vi "Pack PII Error_v00.vi"(8 "PII+Error Doubler":T4, 9 "PII+Error MCC":T4, 10 "PII+Error B":T4, 11 "PII+Error A":T4) -> (0 "Thresholds":T1, 3 "Error packed":T3={"Pre-Offset"={"Pre-Offset 1"=2, "Pre-Offset 2"=0, "Pre-Offset 3"=0, "Pre-Offset 4"=0, "Pre-Offset 5"=2, "Pre-Offset 6"=0, "Pre-Offset 7"=0, "Pre-Offset 8"=0}, "Post-Offset "={"Offset 1"=0, "Offset 2"=0, "Offset 3"=0, "Offset 4"=0, "Offset 5"=0, "Offset 6"=0, "Offset 7"=0, "Offset 8"=0}, "Gains"={"Gain 1"=0, "Gain 2"=0, "Gain 3"=0, "Gain 4"=0, "Gain 5"=0, "Gain 6"=0, "Gain 7"=0, "Gain 8"=0}, "Polarity DC"={"False 1"=FALSE, "False 2"=FALSE, "False 3"=FALSE, "False 4"=FALSE, "DC x -1"=FALSE, "DC x -1 2"=FALSE, "DC x -1 3"=FALSE, "DC x -1 4"=FALSE}})   [LabVIEW 2010]
doc: "Packages individual values related to error signal scaling from the user interface into data structures compatible with FPGA_Cavities.VI\n(very messy, could use a tidy)."
uses:
  Strict Type Defs/Error Scale.ctl
  Strict Type Defs/Controls Converted.ctl
  Strict Type Defs/Errors Converted.ctl
  Strict Type Defs/PII individual.ctl
panel:
  in  "Thresholds type def":T1
  in  "Re-Scan Thresh":T2
  in  "Lock Thresh":T2
  in  "Error scale FPGA type def":T3={"Pre-Offset"={"Pre-Offset 1"=0, "Pre-Offset 2"=300, "Pre-Offset 3"=0, "Pre-Offset 4"=0, "Pre-Offset 5"=0, "Pre-Offset 6"=0, "Pre-Offset 7"=0, "Pre-Offset 8"=0}, "Post-Offset "={"Offset 1"=0, "Offset 2"=300, "Offset 3"=0, "Offset 4"=0, "Offset 5"=0, "Offset 6"=0, "Offset 7"=0, "Offset 8"=0}, "Gains"={"Gain 1"=1, "Gain 2"=1, "Gain 3"=1, "Gain 4"=1, "Gain 5"=1, "Gain 6"=1, "Gain 7"=1, "Gain 8"=1}, "Polarity DC"={"False 1"=FALSE, "False 2"=FALSE, "False 3"=FALSE, "False 4"=FALSE, "DC x -1"=FALSE, "DC x -1 2"=FALSE, "DC x -1 3"=FALSE, "DC x -1 4"=FALSE}}
  in  "Polarity DC":T7
  in  "Pre Offset":T8
  in  "Offset":T9
  in  "Gains":T10
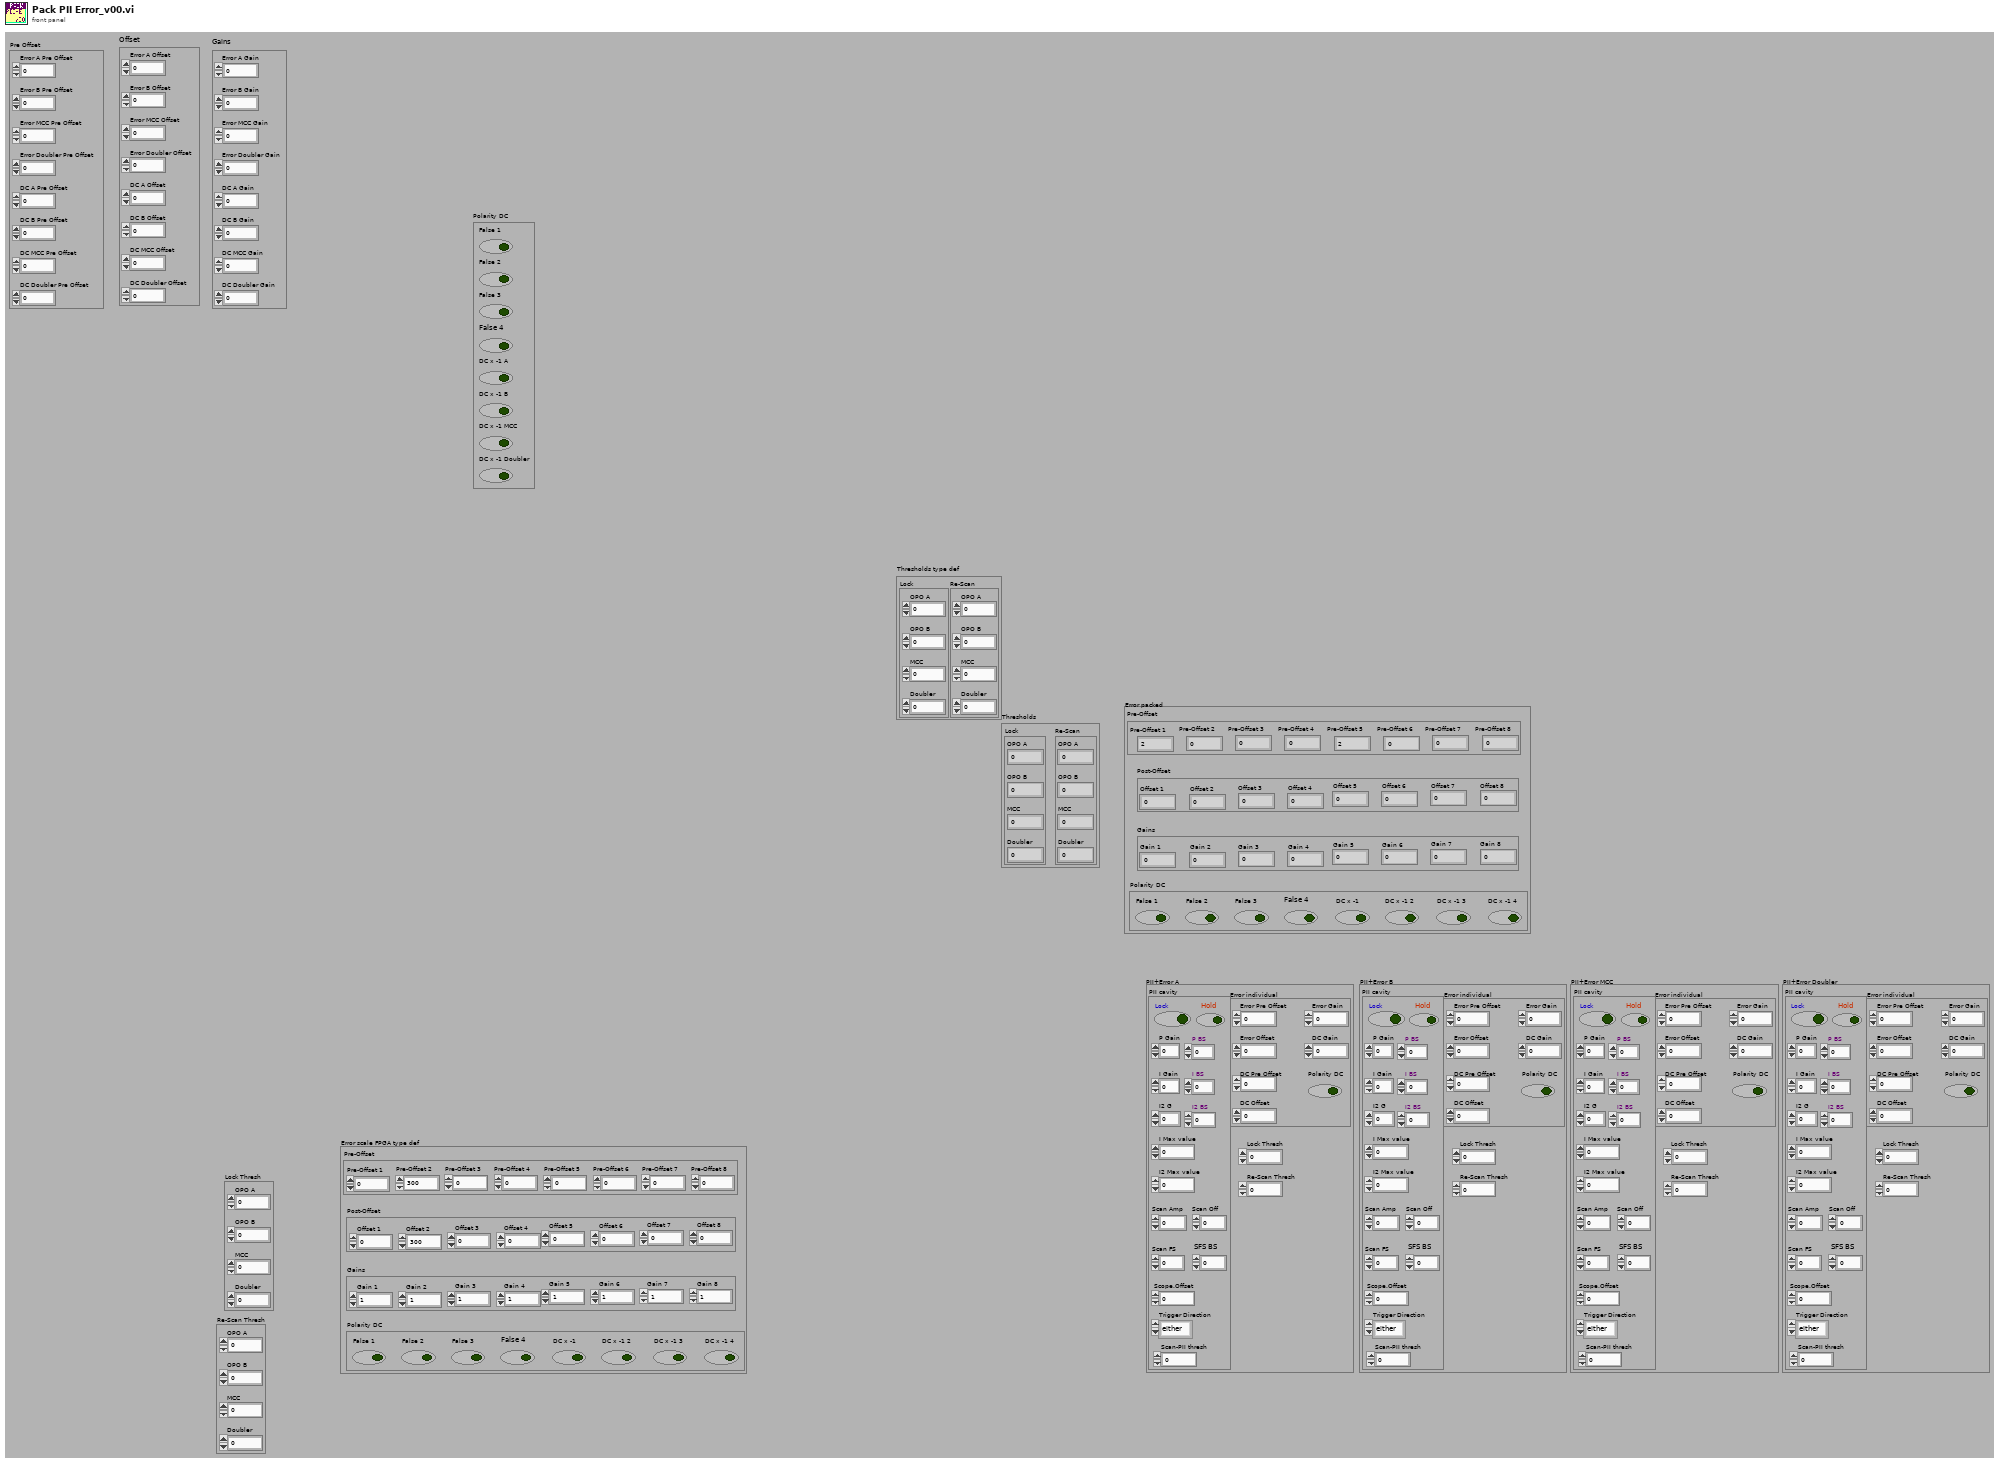
[diagram p1: front panel]
types:
  T1 = cluster{"Lock":cluster{"OPO A":i16, "OPO B":i16, "MCC":i16, "Doubler":i16}, "Re-Scan":cluster{"OPO A":i16, "OPO B":i16, "MCC":i16, "Doubler":i16}}
  T2 = cluster{"OPO A":i16, "OPO B":i16, "MCC":i16, "Doubler":i16}
  T3 = typedef "Error Scale.ctl" = cluster{"Pre-Offset":cluster{"Pre-Offset 1":i16, "Pre-Offset 2":i16, "Pre-Offset 3":i16, "Pre-Offset 4":i16, "Pre-Offset 5":i16, "Pre-Offset 6":i16, "Pre-Offset 7":i16, "Pre-Offset 8":i16}, "Post-Offset ":cluster{"Offset 1":i16, "Offset 2":i16, "Offset 3":i16, "Offset 4":i16, "Offset 5":i16, "Offset 6":i16, "Offset 7":i16, "Offset 8":i16}, "Gains":cluster{"Gain 1":i16, "Gain 2":i16, "Gain 3":i16, "Gain 4":i16, "Gain 5":i16, "Gain 6":i16, "Gain 7":i16, "Gain 8":i16}, "Polarity DC":cluster{"False 1":bool, "False 2":bool, "False 3":bool, "False 4":bool, "DC x -1":bool, "DC x -1 2":bool, "DC x -1 3":bool, "DC x -1 4":bool}}
  T4 = typedef "Controls Converted.ctl" = cluster{"Error individual":T5, "PII cavity":T6, "Lock Thresh":i16, "Re-Scan Thresh":i16}
  T5 = typedef "Errors Converted.ctl" = cluster{"Error Pre Offset":i16, "Error Offset":i16, "DC Pre Offset":i16, "DC Offset":i16, "Polarity DC":bool, "Error Gain":i16, "DC Gain":i16}
  T6 = typedef "PII individual.ctl" = cluster{"Lock":bool, "Hold":bool, "P Gain":i32, "P BS":i16, "I Gain":i32, "I BS":i16, "I2 G":i32, "I2 BS":i16, "Scan Amp":i16, "Scan Off":i16, "Scan FS":u16, "SFS BS":i16, "I Max value":i32, "I2 Max value":i32, "Scope.Offset":i16, "Trigger Direction":enum8{"either", "minus-plus", "plus-minus"}, "Scan-PII thresh":i16}
  T7 = cluster{"False 1":bool, "False 2":bool, "False 3":bool, "False 4":bool, "DC x -1 A":bool, "DC x -1 B":bool, "DC x -1 MCC":bool, "DC x -1 Doubler":bool}
  T8 = cluster{"Error A Pre Offset":i16, "Error B Pre Offset":i16, "Error MCC Pre Offset":i16, "Error Doubler Pre Offset":i16, "DC A Pre Offset":i16, "DC B Pre Offset":i16, "DC MCC Pre Offset":i16, "DC Doubler Pre Offset":i16}
  T9 = cluster{"Error A Offset":i16, "Error B Offset":i16, "Error MCC Offset":i16, "Error Doubler Offset":i16, "DC A Offset":i16, "DC B Offset":i16, "DC MCC Offset":i16, "DC Doubler Offset":i16}
  T10 = cluster{"Error A Gain":i16, "Error B Gain":i16, "Error MCC Gain":i16, "Error Doubler Gain":i16, "DC A Gain":i16, "DC B Gain":i16, "DC MCC Gain":i16, "DC Doubler Gain":i16}
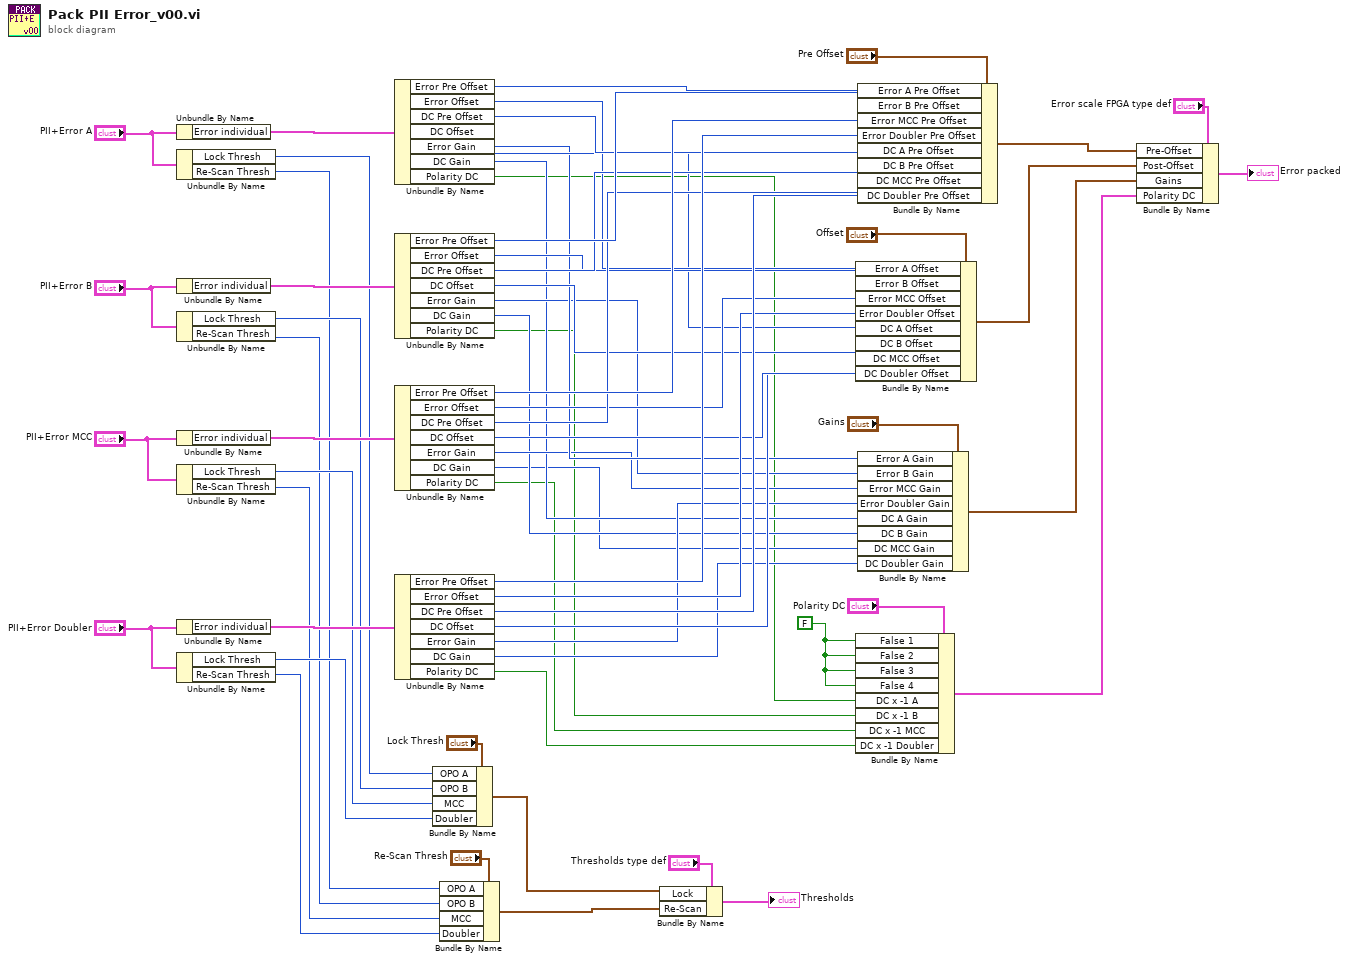
[diagram p0: block diagram]
diagram:
  w27 = FALSE ("False 1")
  n1 = Unbundle By Name("PII+Error A") -> ("Error individual"=w60:T5)
  n2 = Unbundle By Name("PII+Error A") -> ("Lock Thresh"=w13:i16, "Re-Scan Thresh"=w8:i16)
  n3 = Unbundle By Name("PII+Error B") -> ("Error individual"=w59:T5)
  n4 = Unbundle By Name("PII+Error B") -> ("Lock Thresh"=w12:i16, "Re-Scan Thresh"=w7:i16)
  n5 = Unbundle By Name("PII+Error MCC") -> ("Error individual"=w57:T5)
  n6 = Unbundle By Name("PII+Error MCC") -> ("Lock Thresh"=w11:i16, "Re-Scan Thresh"=w6:i16)
  n7 = Unbundle By Name("PII+Error Doubler") -> ("Error individual"=w58:T5)
  n8 = Unbundle By Name("PII+Error Doubler") -> ("Lock Thresh"=w10:i16, "Re-Scan Thresh"=w5:i16)
  n9 = Unbundle By Name(w60) -> ("Error Pre Offset"=w55:i16, "Error Offset"=w47:i16, "DC Pre Offset"=w51:i16, "DC Offset"=w43:i16, "Error Gain"=w39:i16, "DC Gain"=w35:i16, "Polarity DC"=w31:bool)
  n10 = Unbundle By Name(w59) -> ("Error Pre Offset"=w54:i16, "Error Offset"=w46:i16, "DC Pre Offset"=w50:i16, "DC Offset"=w42:i16, "Error Gain"=w38:i16, "DC Gain"=w34:i16, "Polarity DC"=w30:bool)
  n11 = Unbundle By Name(w57) -> ("Error Pre Offset"=w53:i16, "Error Offset"=w45:i16, "DC Pre Offset"=w49:i16, "DC Offset"=w41:i16, "Error Gain"=w37:i16, "DC Gain"=w33:i16, "Polarity DC"=w29:bool)
  n12 = Unbundle By Name(w58) -> ("Error Pre Offset"=w52:i16, "Error Offset"=w44:i16, "DC Pre Offset"=w48:i16, "DC Offset"=w40:i16, "Error Gain"=w36:i16, "DC Gain"=w32:i16, "Polarity DC"=w28:bool)
  n13 = Bundle By Name(cluster="Lock Thresh", "OPO A"=w13, "OPO B"=w12, "MCC"=w11, "Doubler"=w10) -> (w3:T2)
  n14 = Bundle By Name(cluster="Re-Scan Thresh", "OPO A"=w8, "OPO B"=w7, "MCC"=w6, "Doubler"=w5) -> (w2:T2)
  n15 = Bundle By Name(cluster="Thresholds type def", "Lock"=w3, "Re-Scan"=w2) -> (→"Thresholds":T1)
  n16 = Bundle By Name(cluster="Offset", "Error A Offset"=w47, "Error B Offset"=w46, "Error MCC Offset"=w45, "Error Doubler Offset"=w44, "DC A Offset"=w43, "DC B Offset"=w42, "DC MCC Offset"=w41, "DC Doubler Offset"=w40) -> (w16:T9)
  n17 = Bundle By Name(cluster="Polarity DC", "False 1"=w27, "False 2"=w27, "False 3"=w27, "False 4"=w27, "DC x -1 A"=w31, "DC x -1 B"=w30, "DC x -1 MCC"=w29, "DC x -1 Doubler"=w28) -> (w25:T7)
  n18 = Bundle By Name(cluster="Pre Offset", "Error A Pre Offset"=w55, "Error B Pre Offset"=w54, "Error MCC Pre Offset"=w53, "Error Doubler Pre Offset"=w52, "DC A Pre Offset"=w51, "DC B Pre Offset"=w50, "DC MCC Pre Offset"=w49, "DC Doubler Pre Offset"=w48) -> (w26:T8)
  n19 = Bundle By Name(cluster="Gains", "Error A Gain"=w39, "Error B Gain"=w38, "Error MCC Gain"=w37, "Error Doubler Gain"=w36, "DC A Gain"=w35, "DC B Gain"=w34, "DC MCC Gain"=w33, "DC Doubler Gain"=w32) -> (w18:T10)
  n20 = Bundle By Name(cluster="Error scale FPGA type def", "Pre-Offset"=w26, "Post-Offset"=w16, "Gains"=w18, "Polarity DC"=w25) -> (→"Error packed":T3)
